vi "Read Msg Input.vi"(11 "Stopped Msg Input in":refnum<class "Stopped Msg Input.lvclass">) -> (1 "Error":errorcluster, 2 "Unified Actor":refnum<class "Actor.lvclass">, 4 "Teller":refnum<class "Teller.lvclass">)   [LabVIEW 2020, in "jettl.lvlib" / "Stopped jettl Msg.lvlib" / "Stopped Msg Input.lvlib" / "Stopped Msg Input.lvclass"]
uses:
  Stopped Msg Input.lvclass
  Actor/Actor.lvclass
  Teller/Teller.lvclass
  Stopped Msg Input.lvclass/Stopped Msg Input.ctl
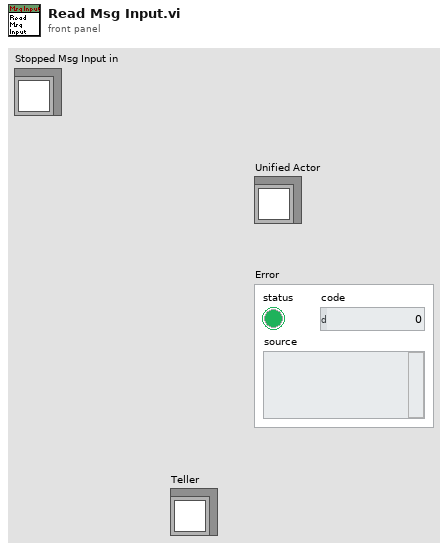
[diagram p1: front panel]
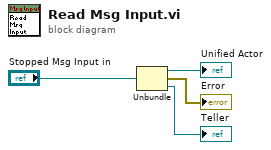
[diagram p0: block diagram]
diagram:
  n1 = Unbundle "Unbundle"("Stopped Msg Input in") -> (→"Unified Actor":refnum<class "Actor.lvclass">, →"Error":errorcluster, →"Teller":refnum<class "Teller.lvclass">)
